vi "del2.vi"() -> ()   [LabVIEW 2025]
uses:
  Table_Filtering/Table_Filtering.lvlib
panel:
  in  "stop":bool
  out "Dataframe":string[][](array[string])
  out "Packets":string[][](table)=[["10", "11/14/2025 1:57:47 PM", "10.0.0.1", "10.0.0.2", "UDP", "0.821211", "thisisdata"], ["100", "11/14/2025 1:57:47 PM", "10.0.0.1", "10.0.0.2", "UDP", "0.956516", "thisisdata"], ["1002", "11/14/2025 1:57:47 PM", "10.0.0.1", "10.0.0.2", "UDP", "0.960987", "thisisdata"], ["1007", "11/14/2025 1:57:47 PM", "10.0.0.1", "10.0.0.2", "UDP", "0.867598", "thisisdata"], ["1009", "11/14/2025 1:57:47 PM", "10.0.0.1", "10.0.0.2", "UDP", "0.839638", "thisisdata"], ["101", "11/14/2025 1:57:47 PM", "10.0.0.1", "10.0.0.2", "UDP", "0.891709", "thisisdata"], ["1012", "11/14/2025 1:57:47 PM", "10.0.0.1", "10.0.0.2", "UDP", "0.969576", "thisisdata"], ["1017", "11/14/2025 1:57:47 PM", "10.0.0.1", "10.0.0.2", "UDP", "0.871748", "thisisdata"], ["1021", "11/14/2025 1:57:47 PM", "10.0.0.1", "10.0.0.2", "UDP", "0.904588", "thisisdata"], ["1026", "11/14/2025 1:57:47 PM", "10.0.0.1", "10.0.0.2", "UDP", "0.986150", "thisisdata"], ["1027", "11/14/2025 1:57:47 PM", "10.0.0.1", "10.0.0.2", "UDP", "0.775009", "thisisdata"], ["1028", "11/14/2025 1:57:47 PM", "10.0.0.1", "10.0.0.2", "UDP", "0.817026", "thisisdata"], ["1036", "11/14/2025 1:57:47 PM", "10.0.0.1", "10.0.0.2", "UDP", "0.839495", "thisisdata"], ["1038", "11/14/2025 1:57:47 PM", "10.0.0.1", "10.0.0.2", "UDP", "0.847314", "thisisdata"], ["1044", "11/14/2025 1:57:47 PM", "10.0.0.1", "10.0.0.2", "UDP", "0.793260", "thisisdata"], ["1048", "11/14/2025 1:57:47 PM", "10.0.0.1", "10.0.0.2", "UDP", "0.742047", "thisisdata"], ["1049", "11/14/2025 1:57:47 PM", "10.0.0.1", "10.0.0.2", "UDP", "0.771430", "thisisdata"], ["1051", "11/14/2025 1:57:47 PM", "10.0.0.1", "10.0.0.2", "UDP", "0.889463", "thisisdata"], ["1052", "11/14/2025 1:57:47 PM", "10.0.0.1", "10.0.0.2", "UDP", "0.702476", "thisisdata"], ["1053", "11/14/2025 1:57:47 PM", "10.0.0.1", "10.0.0.2", "UDP", "0.943543", "thisisdata"], ["1055", "11/14/2025 1:57:47 PM", "10.0.0.1", "10.0.0.2", "UDP", "0.912358", "thisisdata"], ["1062", "11/14/2025 1:57:47 PM", "10.0.0.1", "10.0.0.2", "UDP", "0.883876", "thisisdata"], ["1065", "11/14/2025 1:57:47 PM", "10.0.0.1", "10.0.0.2", "UDP", "0.998758", "thisisdata"], ["1066", "11/14/2025 1:57:47 PM", "10.0.0.1", "10.0.0.2", "UDP", "0.980816", "thisisdata"], ["1067", "11/14/2025 1:57:47 PM", "10.0.0.1", "10.0.0.2", "UDP", "0.862874", "thisisdata"], ["1074", "11/14/2025 1:57:47 PM", "10.0.0.1", "10.0.0.2", "UDP", "0.985200", "thisisdata"], ["1075", "11/14/2025 1:57:47 PM", "10.0.0.1", "10.0.0.2", "UDP", "0.895925", "thisisdata"], ["108", "11/14/2025 1:57:47 PM", "10.0.0.1", "10.0.0.2", "UDP", "0.746068", "thisisdata"], ["1083", "11/14/2025 1:57:47 PM", "10.0.0.1", "10.0.0.2", "UDP", "0.976636", "thisisdata"], ["1084", "11/14/2025 1:57:47 PM", "10.0.0.1", "10.0.0.2", "UDP", "0.746952", "thisisdata"], ["1086", "11/14/2025 1:57:47 PM", "10.0.0.1", "10.0.0.2", "UDP", "0.772755", "thisisdata"], ["1088", "11/14/2025 1:57:47 PM", "10.0.0.1", "10.0.0.2", "UDP", "0.942784", "thisisdata"], ["1090", "11/14/2025 1:57:47 PM", "10.0.0.1", "10.0.0.2", "UDP", "0.927067", "thisisdata"], ["1092", "11/14/2025 1:57:47 PM", "10.0.0.1", "10.0.0.2", "UDP", "0.875037", "thisisdata"], ["11", "11/14/2025 1:57:47 PM", "10.0.0.1", "10.0.0.2", "UDP", "0.939175", "thisisdata"], ["1101", "11/14/2025 1:57:47 PM", "10.0.0.1", "10.0.0.2", "UDP", "0.730371", "thisisdata"], ["1102", "11/14/2025 1:57:47 PM", "10.0.0.1", "10.0.0.2", "UDP", "0.711041", "thisisdata"], ["1103", "11/14/2025 1:57:47 PM", "10.0.0.1", "10.0.0.2", "UDP", "0.802089", "thisisdata"], ["1104", "11/14/2025 1:57:47 PM", "10.0.0.1", "10.0.0.2", "UDP", "0.975316", "thisisdata"], ["1108", "11/14/2025 1:57:47 PM", "10.0.0.1", "10.0.0.2", "UDP", "0.840307", "thisisdata"], ["1111", "11/14/2025 1:57:47 PM", "10.0.0.1", "10.0.0.2", "UDP", "0.734069", "thisisdata"], ["1113", "11/14/2025 1:57:47 PM", "10.0.0.1", "10.0.0.2", "UDP", "0.897764", "thisisdata"], ["1114", "11/14/2025 1:57:47 PM", "10.0.0.1", "10.0.0.2", "UDP", "0.704577", "thisisdata"], ["1115", "11/14/2025 1:57:47 PM", "10.0.0.1", "10.0.0.2", "UDP", "0.831595", "thisisdata"], ["1123", "11/14/2025 1:57:47 PM", "10.0.0.1", "10.0.0.2", "UDP", "0.869848", "thisisdata"], ["1130", "11/14/2025 1:57:47 PM", "10.0.0.1", "10.0.0.2", "UDP", "0.848458", "thisisdata"], ["1131", "11/14/2025 1:57:47 PM", "10.0.0.1", "10.0.0.2", "UDP", "0.914476", "thisisdata"], ["1139", "11/14/2025 1:57:47 PM", "10.0.0.1", "10.0.0.2", "UDP", "0.851881", "thisisdata"], ["1142", "11/14/2025 1:57:47 PM", "10.0.0.1", "10.0.0.2", "UDP", "0.781918", "thisisdata"], ["1148", "11/14/2025 1:57:47 PM", "10.0.0.1", "10.0.0.2", "UDP", "0.839308", "thisisdata"], ["115", "11/14/2025 1:57:47 PM", "10.0.0.1", "10.0.0.2", "UDP", "0.824463", "thisisdata"], ["1153", "11/14/2025 1:57:47 PM", "10.0.0.1", "10.0.0.2", "UDP", "0.762073", "thisisdata"], ["116", "11/14/2025 1:57:47 PM", "10.0.0.1", "10.0.0.2", "UDP", "0.718284", "thisisdata"], ["1164", "11/14/2025 1:57:47 PM", "10.0.0.1", "10.0.0.2", "UDP", "0.901802", "thisisdata"], ["1165", "11/14/2025 1:57:47 PM", "10.0.0.1", "10.0.0.2", "UDP", "0.782467", "thisisdata"], ["1168", "11/14/2025 1:57:47 PM", "10.0.0.1", "10.0.0.2", "UDP", "0.901873", "thisisdata"], ["1177", "11/14/2025 1:57:47 PM", "10.0.0.1", "10.0.0.2", "UDP", "0.889595", "thisisdata"], ["118", "11/14/2025 1:57:47 PM", "10.0.0.1", "10.0.0.2", "UDP", "0.966309", "thisisdata"], ["1181", "11/14/2025 1:57:47 PM", "10.0.0.1", "10.0.0.2", "UDP", "0.741139", "thisisdata"], ["1182", "11/14/2025 1:57:47 PM", "10.0.0.1", "10.0.0.2", "UDP", "0.954023", "thisisdata"], ["1183", "11/14/2025 1:57:47 PM", "10.0.0.1", "10.0.0.2", "UDP", "0.881562", "thisisdata"], ["1184", "11/14/2025 1:57:47 PM", "10.0.0.1", "10.0.0.2", "UDP", "0.852993", "thisisdata"], ["1185", "11/14/2025 1:57:47 PM", "10.0.0.1", "10.0.0.2", "UDP", "0.885773", "thisisdata"], ["1187", "11/14/2025 1:57:47 PM", "10.0.0.1", "10.0.0.2", "UDP", "0.801737", "thisisdata"], ["1195", "11/14/2025 1:57:47 PM", "10.0.0.1", "10.0.0.2", "UDP", "0.790347", "thisisdata"], ["1196", "11/14/2025 1:57:47 PM", "10.0.0.1", "10.0.0.2", "UDP", "0.864754", "thisisdata"], ["1197", "11/14/2025 1:57:47 PM", "10.0.0.1", "10.0.0.2", "UDP", "0.709221", "thisisdata"], ["121", "11/14/2025 1:57:47 PM", "10.0.0.1", "10.0.0.2", "UDP", "0.913497", "thisisdata"], ["1211", "11/14/2025 1:57:47 PM", "10.0.0.1", "10.0.0.2", "UDP", "0.965122", "thisisdata"], ["1213", "11/14/2025 1:57:47 PM", "10.0.0.1", "10.0.0.2", "UDP", "0.973075", "thisisdata"], ["1218", "11/14/2025 1:57:47 PM", "10.0.0.1", "10.0.0.2", "UDP", "0.904226", "thisisdata"], ["1222", "11/14/2025 1:57:47 PM", "10.0.0.1", "10.0.0.2", "UDP", "0.828121", "thisisdata"], ["1225", "11/14/2025 1:57:47 PM", "10.0.0.1", "10.0.0.2", "UDP", "0.730012", "thisisdata"], ["1226", "11/14/2025 1:57:47 PM", "10.0.0.1", "10.0.0.2", "UDP", "0.762505", "thisisdata"], ["123", "11/14/2025 1:57:47 PM", "10.0.0.1", "10.0.0.2", "UDP", "0.900157", "thisisdata"], ["1230", "11/14/2025 1:57:47 PM", "10.0.0.1", "10.0.0.2", "UDP", "0.958830", "thisisdata"], ["1231", "11/14/2025 1:57:47 PM", "10.0.0.1", "10.0.0.2", "UDP", "0.727490", "thisisdata"], ["1232", "11/14/2025 1:57:47 PM", "10.0.0.1", "10.0.0.2", "UDP", "0.913030", "thisisdata"], ["1234", "11/14/2025 1:57:47 PM", "10.0.0.1", "10.0.0.2", "UDP", "0.711353", "thisisdata"], ["1237", "11/14/2025 1:57:47 PM", "10.0.0.1", "10.0.0.2", "UDP", "0.704839", "thisisdata"], ["1240", "11/14/2025 1:57:47 PM", "10.0.0.1", "10.0.0.2", "UDP", "0.808493", "thisisdata"], ["1241", "11/14/2025 1:57:47 PM", "10.0.0.1", "10.0.0.2", "UDP", "0.750334", "thisisdata"], ["1242", "11/14/2025 1:57:47 PM", "10.0.0.1", "10.0.0.2", "UDP", "0.953795", "thisisdata"], ["1243", "11/14/2025 1:57:47 PM", "10.0.0.1", "10.0.0.2", "UDP", "0.914837", "thisisdata"], ["125", "11/14/2025 1:57:47 PM", "10.0.0.1", "10.0.0.2", "UDP", "0.850827", "thisisdata"], ["1252", "11/14/2025 1:57:47 PM", "10.0.0.1", "10.0.0.2", "UDP", "0.889690", "thisisdata"], ["1253", "11/14/2025 1:57:47 PM", "10.0.0.1", "10.0.0.2", "UDP", "0.800545", "thisisdata"], ["1255", "11/14/2025 1:57:47 PM", "10.0.0.1", "10.0.0.2", "UDP", "0.813802", "thisisdata"], ["1262", "11/14/2025 1:57:47 PM", "10.0.0.1", "10.0.0.2", "UDP", "0.882839", "thisisdata"], ["1265", "11/14/2025 1:57:47 PM", "10.0.0.1", "10.0.0.2", "UDP", "0.898409", "thisisdata"], ["127", "11/14/2025 1:57:47 PM", "10.0.0.1", "10.0.0.2", "UDP", "0.713807", "thisisdata"], ["1275", "11/14/2025 1:57:47 PM", "10.0.0.1", "10.0.0.2", "UDP", "0.972156", "thisisdata"], ["1284", "11/14/2025 1:57:47 PM", "10.0.0.1", "10.0.0.2", "UDP", "0.978269", "thisisdata"], ["1289", "11/14/2025 1:57:47 PM", "10.0.0.1", "10.0.0.2", "UDP", "0.740155", "thisisdata"], ["1299", "11/14/2025 1:57:47 PM", "10.0.0.1", "10.0.0.2", "UDP", "0.953843", "thisisdata"], ["13", "11/14/2025 1:57:47 PM", "10.0.0.1", "10.0.0.2", "UDP", "0.842815", "thisisdata"], ["1301", "11/14/2025 1:57:47 PM", "10.0.0.1", "10.0.0.2", "UDP", "0.879611", "thisisdata"], ["1302", "11/14/2025 1:57:47 PM", "10.0.0.1", "10.0.0.2", "UDP", "0.945983", "thisisdata"], ["1303", "11/14/2025 1:57:47 PM", "10.0.0.1", "10.0.0.2", "UDP", "0.755170", "thisisdata"], ["1307", "11/14/2025 1:57:47 PM", "10.0.0.1", "10.0.0.2", "UDP", "0.773780", "thisisdata"], ["1312", "11/14/2025 1:57:47 PM", "10.0.0.1", "10.0.0.2", "UDP", "0.814087", "thisisdata"], ["1314", "11/14/2025 1:57:47 PM", "10.0.0.1", "10.0.0.2", "UDP", "0.980063", "thisisdata"], ["1317", "11/14/2025 1:57:47 PM", "10.0.0.1", "10.0.0.2", "UDP", "0.829011", "thisisdata"], ["1320", "11/14/2025 1:57:47 PM", "10.0.0.1", "10.0.0.2", "UDP", "0.758120", "thisisdata"], ["1321", "11/14/2025 1:57:47 PM", "10.0.0.1", "10.0.0.2", "UDP", "0.759463", "thisisdata"], ["1322", "11/14/2025 1:57:47 PM", "10.0.0.1", "10.0.0.2", "UDP", "0.824116", "thisisdata"], ["1323", "11/14/2025 1:57:47 PM", "10.0.0.1", "10.0.0.2", "UDP", "0.762172", "thisisdata"], ["1324", "11/14/2025 1:57:47 PM", "10.0.0.1", "10.0.0.2", "UDP", "0.885589", "thisisdata"], ["1330", "11/14/2025 1:57:47 PM", "10.0.0.1", "10.0.0.2", "UDP", "0.942420", "thisisdata"], ["1333", "11/14/2025 1:57:47 PM", "10.0.0.1", "10.0.0.2", "UDP", "0.798878", "thisisdata"], ["1338", "11/14/2025 1:57:47 PM", "10.0.0.1", "10.0.0.2", "UDP", "0.748441", "thisisdata"], ["134", "11/14/2025 1:57:47 PM", "10.0.0.1", "10.0.0.2", "UDP", "0.739118", "thisisdata"], ["1341", "11/14/2025 1:57:47 PM", "10.0.0.1", "10.0.0.2", "UDP", "0.912641", "thisisdata"], ["1342", "11/14/2025 1:57:47 PM", "10.0.0.1", "10.0.0.2", "UDP", "0.833794", "thisisdata"], ["1346", "11/14/2025 1:57:47 PM", "10.0.0.1", "10.0.0.2", "UDP", "0.938173", "thisisdata"], ["1348", "11/14/2025 1:57:47 PM", "10.0.0.1", "10.0.0.2", "UDP", "0.703225", "thisisdata"], ["1349", "11/14/2025 1:57:47 PM", "10.0.0.1", "10.0.0.2", "UDP", "0.962230", "thisisdata"], ["1351", "11/14/2025 1:57:47 PM", "10.0.0.1", "10.0.0.2", "UDP", "0.923262", "thisisdata"], ["1357", "11/14/2025 1:57:47 PM", "10.0.0.1", "10.0.0.2", "UDP", "0.977014", "thisisdata"], ["1358", "11/14/2025 1:57:47 PM", "10.0.0.1", "10.0.0.2", "UDP", "0.904471", "thisisdata"], ["1360", "11/14/2025 1:57:47 PM", "10.0.0.1", "10.0.0.2", "UDP", "0.840541", "thisisdata"], ["1364", "11/14/2025 1:57:47 PM", "10.0.0.1", "10.0.0.2", "UDP", "0.759527", "thisisdata"], ["1367", "11/14/2025 1:57:47 PM", "10.0.0.1", "10.0.0.2", "UDP", "0.926483", "thisisdata"], ["1369", "11/14/2025 1:57:47 PM", "10.0.0.1", "10.0.0.2", "UDP", "0.897696", "thisisdata"], ["1371", "11/14/2025 1:57:47 PM", "10.0.0.1", "10.0.0.2", "UDP", "0.987694", "thisisdata"], ["1374", "11/14/2025 1:57:47 PM", "10.0.0.1", "10.0.0.2", "UDP", "0.795706", "thisisdata"], ["1377", "11/14/2025 1:57:47 PM", "10.0.0.1", "10.0.0.2", "UDP", "0.927883", "thisisdata"], ["1378", "11/14/2025 1:57:47 PM", "10.0.0.1", "10.0.0.2", "UDP", "0.986175", "thisisdata"], ["1379", "11/14/2025 1:57:47 PM", "10.0.0.1", "10.0.0.2", "UDP", "0.716053", "thisisdata"], ["138", "11/14/2025 1:57:47 PM", "10.0.0.1", "10.0.0.2", "UDP", "0.961495", "thisisdata"], ["1381", "11/14/2025 1:57:47 PM", "10.0.0.1", "10.0.0.2", "UDP", "0.839552", "thisisdata"], ["1382", "11/14/2025 1:57:47 PM", "10.0.0.1", "10.0.0.2", "UDP", "0.914187", "thisisdata"], ["1388", "11/14/2025 1:57:47 PM", "10.0.0.1", "10.0.0.2", "UDP", "0.890783", "thisisdata"], ["1390", "11/14/2025 1:57:47 PM", "10.0.0.1", "10.0.0.2", "UDP", "0.913426", "thisisdata"], ["1391", "11/14/2025 1:57:47 PM", "10.0.0.1", "10.0.0.2", "UDP", "0.758421", "thisisdata"], ["1394", "11/14/2025 1:57:47 PM", "10.0.0.1", "10.0.0.2", "UDP", "0.884168", "thisisdata"], ["1395", "11/14/2025 1:57:47 PM", "10.0.0.1", "10.0.0.2", "UDP", "0.773979", "thisisdata"], ["1397", "11/14/2025 1:57:47 PM", "10.0.0.1", "10.0.0.2", "UDP", "0.827235", "thisisdata"], ["14", "11/14/2025 1:57:47 PM", "10.0.0.1", "10.0.0.2", "UDP", "0.839466", "thisisdata"], ["1403", "11/14/2025 1:57:47 PM", "10.0.0.1", "10.0.0.2", "UDP", "0.889704", "thisisdata"], ["1411", "11/14/2025 1:57:47 PM", "10.0.0.1", "10.0.0.2", "UDP", "0.967881", "thisisdata"], ["1417", "11/14/2025 1:57:47 PM", "10.0.0.1", "10.0.0.2", "UDP", "0.962037", "thisisdata"], ["1418", "11/14/2025 1:57:47 PM", "10.0.0.1", "10.0.0.2", "UDP", "0.951923", "thisisdata"], ["1419", "11/14/2025 1:57:47 PM", "10.0.0.1", "10.0.0.2", "UDP", "0.912131", "thisisdata"], ["142", "11/14/2025 1:57:47 PM", "10.0.0.1", "10.0.0.2", "UDP", "0.900485", "thisisdata"], ["1421", "11/14/2025 1:57:47 PM", "10.0.0.1", "10.0.0.2", "UDP", "0.972293", "thisisdata"], ["1428", "11/14/2025 1:57:47 PM", "10.0.0.1", "10.0.0.2", "UDP", "0.706623", "thisisdata"], ["143", "11/14/2025 1:57:47 PM", "10.0.0.1", "10.0.0.2", "UDP", "0.862774", "thisisdata"], ["1430", "11/14/2025 1:57:47 PM", "10.0.0.1", "10.0.0.2", "UDP", "0.831932", "thisisdata"], ["1432", "11/14/2025 1:57:47 PM", "10.0.0.1", "10.0.0.2", "UDP", "0.955880", "thisisdata"], ["1434", "11/14/2025 1:57:47 PM", "10.0.0.1", "10.0.0.2", "UDP", "0.885487", "thisisdata"], ["1436", "11/14/2025 1:57:47 PM", "10.0.0.1", "10.0.0.2", "UDP", "0.804128", "thisisdata"], ["144", "11/14/2025 1:57:47 PM", "10.0.0.1", "10.0.0.2", "UDP", "0.837449", "thisisdata"], ["1440", "11/14/2025 1:57:47 PM", "10.0.0.1", "10.0.0.2", "UDP", "0.973148", "thisisdata"], ["1447", "11/14/2025 1:57:47 PM", "10.0.0.1", "10.0.0.2", "UDP", "0.718230", "thisisdata"], ["1449", "11/14/2025 1:57:47 PM", "10.0.0.1", "10.0.0.2", "UDP", "0.724932", "thisisdata"], ["145", "11/14/2025 1:57:47 PM", "10.0.0.1", "10.0.0.2", "UDP", "0.834936", "thisisdata"], ["1453", "11/14/2025 1:57:47 PM", "10.0.0.1", "10.0.0.2", "UDP", "0.709100", "thisisdata"], ["1457", "11/14/2025 1:57:47 PM", "10.0.0.1", "10.0.0.2", "UDP", "0.785225", "thisisdata"], ["146", "11/14/2025 1:57:47 PM", "10.0.0.1", "10.0.0.2", "UDP", "0.967161", "thisisdata"], ["1467", "11/14/2025 1:57:47 PM", "10.0.0.1", "10.0.0.2", "UDP", "0.721965", "thisisdata"], ["1468", "11/14/2025 1:57:47 PM", "10.0.0.1", "10.0.0.2", "UDP", "0.994270", "thisisdata"], ["1469", "11/14/2025 1:57:47 PM", "10.0.0.1", "10.0.0.2", "UDP", "0.848087", "thisisdata"], ["147", "11/14/2025 1:57:47 PM", "10.0.0.1", "10.0.0.2", "UDP", "0.777765", "thisisdata"], ["1473", "11/14/2025 1:57:47 PM", "10.0.0.1", "10.0.0.2", "UDP", "0.959502", "thisisdata"], ["1474", "11/14/2025 1:57:47 PM", "10.0.0.1", "10.0.0.2", "UDP", "0.934426", "thisisdata"], ["1475", "11/14/2025 1:57:47 PM", "10.0.0.1", "10.0.0.2", "UDP", "0.755909", "thisisdata"], ["1480", "11/14/2025 1:57:47 PM", "10.0.0.1", "10.0.0.2", "UDP", "0.947402", "thisisdata"], ["1482", "11/14/2025 1:57:47 PM", "10.0.0.1", "10.0.0.2", "UDP", "0.966904", "thisisdata"], ["1488", "11/14/2025 1:57:47 PM", "10.0.0.1", "10.0.0.2", "UDP", "0.717426", "thisisdata"], ["1494", "11/14/2025 1:57:47 PM", "10.0.0.1", "10.0.0.2", "UDP", "0.937831", "thisisdata"], ["1496", "11/14/2025 1:57:47 PM", "10.0.0.1", "10.0.0.2", "UDP", "0.872401", "thisisdata"], ["1497", "11/14/2025 1:57:47 PM", "10.0.0.1", "10.0.0.2", "UDP", "0.814240", "thisisdata"], ["1498", "11/14/2025 1:57:47 PM", "10.0.0.1", "10.0.0.2", "UDP", "0.750281", "thisisdata"], ["151", "11/14/2025 1:57:47 PM", "10.0.0.1", "10.0.0.2", "UDP", "0.875864", "thisisdata"], ["152", "11/14/2025 1:57:47 PM", "10.0.0.1", "10.0.0.2", "UDP", "0.771317", "thisisdata"], ["153", "11/14/2025 1:57:47 PM", "10.0.0.1", "10.0.0.2", "UDP", "0.839422", "thisisdata"], ["156", "11/14/2025 1:57:47 PM", "10.0.0.1", "10.0.0.2", "UDP", "0.729712", "thisisdata"], ["158", "11/14/2025 1:57:47 PM", "10.0.0.1", "10.0.0.2", "UDP", "0.878224", "thisisdata"], ["159", "11/14/2025 1:57:47 PM", "10.0.0.1", "10.0.0.2", "UDP", "0.963331", "thisisdata"], ["16", "11/14/2025 1:57:47 PM", "10.0.0.1", "10.0.0.2", "UDP", "0.706402", "thisisdata"], ["160", "11/14/2025 1:57:47 PM", "10.0.0.1", "10.0.0.2", "UDP", "0.803364", "thisisdata"], ["161", "11/14/2025 1:57:47 PM", "10.0.0.1", "10.0.0.2", "UDP", "0.841035", "thisisdata"], ["162", "11/14/2025 1:57:47 PM", "10.0.0.1", "10.0.0.2", "UDP", "0.815937", "thisisdata"], ["171", "11/14/2025 1:57:47 PM", "10.0.0.1", "10.0.0.2", "UDP", "0.923770", "thisisdata"], ["175", "11/14/2025 1:57:47 PM", "10.0.0.1", "10.0.0.2", "UDP", "0.775138", "thisisdata"], ["182", "11/14/2025 1:57:47 PM", "10.0.0.1", "10.0.0.2", "UDP", "0.769656", "thisisdata"], ["183", "11/14/2025 1:57:47 PM", "10.0.0.1", "10.0.0.2", "UDP", "0.886119", "thisisdata"], ["184", "11/14/2025 1:57:47 PM", "10.0.0.1", "10.0.0.2", "UDP", "0.717707", "thisisdata"], ["186", "11/14/2025 1:57:47 PM", "10.0.0.1", "10.0.0.2", "UDP", "0.963742", "thisisdata"], ["189", "11/14/2025 1:57:47 PM", "10.0.0.1", "10.0.0.2", "UDP", "0.822883", "thisisdata"], ["204", "11/14/2025 1:57:47 PM", "10.0.0.1", "10.0.0.2", "UDP", "0.812997", "thisisdata"], ["211", "11/14/2025 1:57:47 PM", "10.0.0.1", "10.0.0.2", "UDP", "0.819247", "thisisdata"], ["215", "11/14/2025 1:57:47 PM", "10.0.0.1", "10.0.0.2", "UDP", "0.723501", "thisisdata"], ["218", "11/14/2025 1:57:47 PM", "10.0.0.1", "10.0.0.2", "UDP", "0.817730", "thisisdata"], ["222", "11/14/2025 1:57:47 PM", "10.0.0.1", "10.0.0.2", "UDP", "0.952346", "thisisdata"], ["225", "11/14/2025 1:57:47 PM", "10.0.0.1", "10.0.0.2", "UDP", "0.939892", "thisisdata"], ["226", "11/14/2025 1:57:47 PM", "10.0.0.1", "10.0.0.2", "UDP", "0.992709", "thisisdata"], ["235", "11/14/2025 1:57:47 PM", "10.0.0.1", "10.0.0.2", "UDP", "0.941276", "thisisdata"], ["246", "11/14/2025 1:57:47 PM", "10.0.0.1", "10.0.0.2", "UDP", "0.904690", "thisisdata"], ["25", "11/14/2025 1:57:47 PM", "10.0.0.1", "10.0.0.2", "UDP", "0.910103", "thisisdata"], ["251", "11/14/2025 1:57:47 PM", "10.0.0.1", "10.0.0.2", "UDP", "0.720603", "thisisdata"], ["252", "11/14/2025 1:57:47 PM", "10.0.0.1", "10.0.0.2", "UDP", "0.978412", "thisisdata"], ["253", "11/14/2025 1:57:47 PM", "10.0.0.1", "10.0.0.2", "UDP", "0.859802", "thisisdata"], ["257", "11/14/2025 1:57:47 PM", "10.0.0.1", "10.0.0.2", "UDP", "0.706716", "thisisdata"], ["265", "11/14/2025 1:57:47 PM", "10.0.0.1", "10.0.0.2", "UDP", "0.954216", "thisisdata"], ["266", "11/14/2025 1:57:47 PM", "10.0.0.1", "10.0.0.2", "UDP", "0.978586", "thisisdata"], ["268", "11/14/2025 1:57:47 PM", "10.0.0.1", "10.0.0.2", "UDP", "0.728359", "thisisdata"], ["269", "11/14/2025 1:57:47 PM", "10.0.0.1", "10.0.0.2", "UDP", "0.805801", "thisisdata"], ["27", "11/14/2025 1:57:47 PM", "10.0.0.1", "10.0.0.2", "UDP", "0.890670", "thisisdata"], ["270", "11/14/2025 1:57:47 PM", "10.0.0.1", "10.0.0.2", "UDP", "0.730876", "thisisdata"], ["271", "11/14/2025 1:57:47 PM", "10.0.0.1", "10.0.0.2", "UDP", "0.964321", "thisisdata"], ["273", "11/14/2025 1:57:47 PM", "10.0.0.1", "10.0.0.2", "UDP", "0.822445", "thisisdata"], ["280", "11/14/2025 1:57:47 PM", "10.0.0.1", "10.0.0.2", "UDP", "0.805915", "thisisdata"], ["282", "11/14/2025 1:57:47 PM", "10.0.0.1", "10.0.0.2", "UDP", "0.995119", "thisisdata"], ["285", "11/14/2025 1:57:47 PM", "10.0.0.1", "10.0.0.2", "UDP", "0.702493", "thisisdata"], ["287", "11/14/2025 1:57:47 PM", "10.0.0.1", "10.0.0.2", "UDP", "0.895930", "thisisdata"], ["293", "11/14/2025 1:57:47 PM", "10.0.0.1", "10.0.0.2", "UDP", "0.782899", "thisisdata"], ["30", "11/14/2025 1:57:47 PM", "10.0.0.1", "10.0.0.2", "UDP", "0.919602", "thisisdata"], ["302", "11/14/2025 1:57:47 PM", "10.0.0.1", "10.0.0.2", "UDP", "0.702472", "thisisdata"], ["303", "11/14/2025 1:57:47 PM", "10.0.0.1", "10.0.0.2", "UDP", "0.776732", "thisisdata"], ["304", "11/14/2025 1:57:47 PM", "10.0.0.1", "10.0.0.2", "UDP", "0.805126", "thisisdata"], ["305", "11/14/2025 1:57:47 PM", "10.0.0.1", "10.0.0.2", "UDP", "0.974208", "thisisdata"], ["306", "11/14/2025 1:57:47 PM", "10.0.0.1", "10.0.0.2", "UDP", "0.799271", "thisisdata"], ["307", "11/14/2025 1:57:47 PM", "10.0.0.1", "10.0.0.2", "UDP", "0.985518", "thisisdata"], ["310", "11/14/2025 1:57:47 PM", "10.0.0.1", "10.0.0.2", "UDP", "0.995978", "thisisdata"], ["311", "11/14/2025 1:57:47 PM", "10.0.0.1", "10.0.0.2", "UDP", "0.987227", "thisisdata"], ["312", "11/14/2025 1:57:47 PM", "10.0.0.1", "10.0.0.2", "UDP", "0.797511", "thisisdata"], ["314", "11/14/2025 1:57:47 PM", "10.0.0.1", "10.0.0.2", "UDP", "0.838158", "thisisdata"], ["316", "11/14/2025 1:57:47 PM", "10.0.0.1", "10.0.0.2", "UDP", "0.898183", "thisisdata"], ["319", "11/14/2025 1:57:47 PM", "10.0.0.1", "10.0.0.2", "UDP", "0.813462", "thisisdata"], ["320", "11/14/2025 1:57:47 PM", "10.0.0.1", "10.0.0.2", "UDP", "0.725049", "thisisdata"], ["322", "11/14/2025 1:57:47 PM", "10.0.0.1", "10.0.0.2", "UDP", "0.954221", "thisisdata"], ["324", "11/14/2025 1:57:47 PM", "10.0.0.1", "10.0.0.2", "UDP", "0.773913", "thisisdata"], ["330", "11/14/2025 1:57:47 PM", "10.0.0.1", "10.0.0.2", "UDP", "0.846395", "thisisdata"], ["331", "11/14/2025 1:57:47 PM", "10.0.0.1", "10.0.0.2", "UDP", "0.868667", "thisisdata"], ["333", "11/14/2025 1:57:47 PM", "10.0.0.1", "10.0.0.2", "UDP", "0.915934", "thisisdata"], ["335", "11/14/2025 1:57:47 PM", "10.0.0.1", "10.0.0.2", "UDP", "0.744820", "thisisdata"], ["344", "11/14/2025 1:57:47 PM", "10.0.0.1", "10.0.0.2", "UDP", "0.737303", "thisisdata"], ["345", "11/14/2025 1:57:47 PM", "10.0.0.1", "10.0.0.2", "UDP", "0.744197", "thisisdata"], ["347", "11/14/2025 1:57:47 PM", "10.0.0.1", "10.0.0.2", "UDP", "0.816133", "thisisdata"], ["35", "11/14/2025 1:57:47 PM", "10.0.0.1", "10.0.0.2", "UDP", "0.980754", "thisisdata"], ["359", "11/14/2025 1:57:47 PM", "10.0.0.1", "10.0.0.2", "UDP", "0.710696", "thisisdata"], ["36", "11/14/2025 1:57:47 PM", "10.0.0.1", "10.0.0.2", "UDP", "0.821418", "thisisdata"], ["361", "11/14/2025 1:57:47 PM", "10.0.0.1", "10.0.0.2", "UDP", "0.810013", "thisisdata"], ["369", "11/14/2025 1:57:47 PM", "10.0.0.1", "10.0.0.2", "UDP", "0.918693", "thisisdata"], ["373", "11/14/2025 1:57:47 PM", "10.0.0.1", "10.0.0.2", "UDP", "0.860255", "thisisdata"], ["376", "11/14/2025 1:57:47 PM", "10.0.0.1", "10.0.0.2", "UDP", "0.749631", "thisisdata"], ["38", "11/14/2025 1:57:47 PM", "10.0.0.1", "10.0.0.2", "UDP", "0.844976", "thisisdata"], ["383", "11/14/2025 1:57:47 PM", "10.0.0.1", "10.0.0.2", "UDP", "0.800813", "thisisdata"], ["384", "11/14/2025 1:57:47 PM", "10.0.0.1", "10.0.0.2", "UDP", "0.765681", "thisisdata"], ["391", "11/14/2025 1:57:47 PM", "10.0.0.1", "10.0.0.2", "UDP", "0.710353", "thisisdata"], ["392", "11/14/2025 1:57:47 PM", "10.0.0.1", "10.0.0.2", "UDP", "0.798826", "thisisdata"], ["393", "11/14/2025 1:57:47 PM", "10.0.0.1", "10.0.0.2", "UDP", "0.888259", "thisisdata"], ["394", "11/14/2025 1:57:47 PM", "10.0.0.1", "10.0.0.2", "UDP", "0.728993", "thisisdata"], ["406", "11/14/2025 1:57:47 PM", "10.0.0.1", "10.0.0.2", "UDP", "0.924575", "thisisdata"], ["408", "11/14/2025 1:57:47 PM", "10.0.0.1", "10.0.0.2", "UDP", "0.827347", "thisisdata"], ["41", "11/14/2025 1:57:47 PM", "10.0.0.1", "10.0.0.2", "UDP", "0.897112", "thisisdata"], ["412", "11/14/2025 1:57:47 PM", "10.0.0.1", "10.0.0.2", "UDP", "0.823947", "thisisdata"], ["414", "11/14/2025 1:57:47 PM", "10.0.0.1", "10.0.0.2", "UDP", "0.706129", "thisisdata"], ["415", "11/14/2025 1:57:47 PM", "10.0.0.1", "10.0.0.2", "UDP", "0.712052", "thisisdata"], ["42", "11/14/2025 1:57:47 PM", "10.0.0.1", "10.0.0.2", "UDP", "0.984320", "thisisdata"], ["421", "11/14/2025 1:57:47 PM", "10.0.0.1", "10.0.0.2", "UDP", "0.790512", "thisisdata"], ["428", "11/14/2025 1:57:47 PM", "10.0.0.1", "10.0.0.2", "UDP", "0.825226", "thisisdata"], ["431", "11/14/2025 1:57:47 PM", "10.0.0.1", "10.0.0.2", "UDP", "0.866616", "thisisdata"], ["433", "11/14/2025 1:57:47 PM", "10.0.0.1", "10.0.0.2", "UDP", "0.906895", "thisisdata"], ["442", "11/14/2025 1:57:47 PM", "10.0.0.1", "10.0.0.2", "UDP", "0.885974", "thisisdata"], ["448", "11/14/2025 1:57:47 PM", "10.0.0.1", "10.0.0.2", "UDP", "0.888818", "thisisdata"], ["453", "11/14/2025 1:57:47 PM", "10.0.0.1", "10.0.0.2", "UDP", "0.742889", "thisisdata"], ["456", "11/14/2025 1:57:47 PM", "10.0.0.1", "10.0.0.2", "UDP", "0.808371", "thisisdata"], ["459", "11/14/2025 1:57:47 PM", "10.0.0.1", "10.0.0.2", "UDP", "0.878908", "thisisdata"], ["461", "11/14/2025 1:57:47 PM", "10.0.0.1", "10.0.0.2", "UDP", "0.935594", "thisisdata"], ["463", "11/14/2025 1:57:47 PM", "10.0.0.1", "10.0.0.2", "UDP", "0.917788", "thisisdata"], ["465", "11/14/2025 1:57:47 PM", "10.0.0.1", "10.0.0.2", "UDP", "0.924728", "thisisdata"], ["467", "11/14/2025 1:57:47 PM", "10.0.0.1", "10.0.0.2", "UDP", "0.802965", "thisisdata"], ["471", "11/14/2025 1:57:47 PM", "10.0.0.1", "10.0.0.2", "UDP", "0.920198", "thisisdata"], ["473", "11/14/2025 1:57:47 PM", "10.0.0.1", "10.0.0.2", "UDP", "0.712752", "thisisdata"], ["48", "11/14/2025 1:57:47 PM", "10.0.0.1", "10.0.0.2", "UDP", "0.894854", "thisisdata"], ["484", "11/14/2025 1:57:47 PM", "10.0.0.1", "10.0.0.2", "UDP", "0.934918", "thisisdata"], ["487", "11/14/2025 1:57:47 PM", "10.0.0.1", "10.0.0.2", "UDP", "0.753021", "thisisdata"], ["489", "11/14/2025 1:57:47 PM", "10.0.0.1", "10.0.0.2", "UDP", "0.794461", "thisisdata"], ["493", "11/14/2025 1:57:47 PM", "10.0.0.1", "10.0.0.2", "UDP", "0.879307", "thisisdata"], ["494", "11/14/2025 1:57:47 PM", "10.0.0.1", "10.0.0.2", "UDP", "0.821176", "thisisdata"], ["496", "11/14/2025 1:57:47 PM", "10.0.0.1", "10.0.0.2", "UDP", "0.808411", "thisisdata"], ["498", "11/14/2025 1:57:47 PM", "10.0.0.1", "10.0.0.2", "UDP", "0.911798", "thisisdata"], ["5", "11/14/2025 1:57:47 PM", "10.0.0.1", "10.0.0.2", "UDP", "0.924127", "thisisdata"], ["501", "11/14/2025 1:57:47 PM", "10.0.0.1", "10.0.0.2", "UDP", "0.946039", "thisisdata"], ["505", "11/14/2025 1:57:47 PM", "10.0.0.1", "10.0.0.2", "UDP", "0.800570", "thisisdata"], ["509", "11/14/2025 1:57:47 PM", "10.0.0.1", "10.0.0.2", "UDP", "0.879202", "thisisdata"], ["511", "11/14/2025 1:57:47 PM", "10.0.0.1", "10.0.0.2", "UDP", "0.707965", "thisisdata"], ["517", "11/14/2025 1:57:47 PM", "10.0.0.1", "10.0.0.2", "UDP", "0.759952", "thisisdata"], ["518", "11/14/2025 1:57:47 PM", "10.0.0.1", "10.0.0.2", "UDP", "0.720618", "thisisdata"], ["520", "11/14/2025 1:57:47 PM", "10.0.0.1", "10.0.0.2", "UDP", "0.806107", "thisisdata"], ["530", "11/14/2025 1:57:47 PM", "10.0.0.1", "10.0.0.2", "UDP", "0.995294", "thisisdata"], ["531", "11/14/2025 1:57:47 PM", "10.0.0.1", "10.0.0.2", "UDP", "0.734341", "thisisdata"], ["538", "11/14/2025 1:57:47 PM", "10.0.0.1", "10.0.0.2", "UDP", "0.791430", "thisisdata"], ["552", "11/14/2025 1:57:47 PM", "10.0.0.1", "10.0.0.2", "UDP", "0.803719", "thisisdata"], ["553", "11/14/2025 1:57:47 PM", "10.0.0.1", "10.0.0.2", "UDP", "0.798672", "thisisdata"], ["555", "11/14/2025 1:57:47 PM", "10.0.0.1", "10.0.0.2", "UDP", "0.718180", "thisisdata"], ["556", "11/14/2025 1:57:47 PM", "10.0.0.1", "10.0.0.2", "UDP", "0.712425", "thisisdata"], ["557", "11/14/2025 1:57:47 PM", "10.0.0.1", "10.0.0.2", "UDP", "0.839688", "thisisdata"], ["561", "11/14/2025 1:57:47 PM", "10.0.0.1", "10.0.0.2", "UDP", "0.973886", "thisisdata"], ["575", "11/14/2025 1:57:47 PM", "10.0.0.1", "10.0.0.2", "UDP", "0.829130", "thisisdata"], ["576", "11/14/2025 1:57:47 PM", "10.0.0.1", "10.0.0.2", "UDP", "0.725344", "thisisdata"], ["579", "11/14/2025 1:57:47 PM", "10.0.0.1", "10.0.0.2", "UDP", "0.857040", "thisisdata"], ["580", "11/14/2025 1:57:47 PM", "10.0.0.1", "10.0.0.2", "UDP", "0.919608", "thisisdata"], ["584", "11/14/2025 1:57:47 PM", "10.0.0.1", "10.0.0.2", "UDP", "0.875136", "thisisdata"], ["585", "11/14/2025 1:57:47 PM", "10.0.0.1", "10.0.0.2", "UDP", "0.791057", "thisisdata"], ["59", "11/14/2025 1:57:47 PM", "10.0.0.1", "10.0.0.2", "UDP", "0.836493", "thisisdata"], ["591", "11/14/2025 1:57:47 PM", "10.0.0.1", "10.0.0.2", "UDP", "0.861319", "thisisdata"], ["592", "11/14/2025 1:57:47 PM", "10.0.0.1", "10.0.0.2", "UDP", "0.916902", "thisisdata"], ["599", "11/14/2025 1:57:47 PM", "10.0.0.1", "10.0.0.2", "UDP", "0.903742", "thisisdata"], ["60", "11/14/2025 1:57:47 PM", "10.0.0.1", "10.0.0.2", "UDP", "0.871553", "thisisdata"], ["603", "11/14/2025 1:57:47 PM", "10.0.0.1", "10.0.0.2", "UDP", "0.905091", "thisisdata"], ["606", "11/14/2025 1:57:47 PM", "10.0.0.1", "10.0.0.2", "UDP", "0.886018", "thisisdata"], ["609", "11/14/2025 1:57:47 PM", "10.0.0.1", "10.0.0.2", "UDP", "0.710266", "thisisdata"], ["610", "11/14/2025 1:57:47 PM", "10.0.0.1", "10.0.0.2", "UDP", "0.785021", "thisisdata"], ["614", "11/14/2025 1:57:47 PM", "10.0.0.1", "10.0.0.2", "UDP", "0.714634", "thisisdata"], ["622", "11/14/2025 1:57:47 PM", "10.0.0.1", "10.0.0.2", "UDP", "0.912282", "thisisdata"], ["624", "11/14/2025 1:57:47 PM", "10.0.0.1", "10.0.0.2", "UDP", "0.890598", "thisisdata"], ["631", "11/14/2025 1:57:47 PM", "10.0.0.1", "10.0.0.2", "UDP", "0.748006", "thisisdata"], ["634", "11/14/2025 1:57:47 PM", "10.0.0.1", "10.0.0.2", "UDP", "0.791920", "thisisdata"], ["64", "11/14/2025 1:57:47 PM", "10.0.0.1", "10.0.0.2", "UDP", "0.967066", "thisisdata"], ["642", "11/14/2025 1:57:47 PM", "10.0.0.1", "10.0.0.2", "UDP", "0.783278", "thisisdata"], ["644", "11/14/2025 1:57:47 PM", "10.0.0.1", "10.0.0.2", "UDP", "0.893851", "thisisdata"], ["65", "11/14/2025 1:57:47 PM", "10.0.0.1", "10.0.0.2", "UDP", "0.809766", "thisisdata"], ["657", "11/14/2025 1:57:47 PM", "10.0.0.1", "10.0.0.2", "UDP", "0.710376", "thisisdata"], ["660", "11/14/2025 1:57:47 PM", "10.0.0.1", "10.0.0.2", "UDP", "0.897561", "thisisdata"], ["661", "11/14/2025 1:57:47 PM", "10.0.0.1", "10.0.0.2", "UDP", "0.907407", "thisisdata"], ["668", "11/14/2025 1:57:47 PM", "10.0.0.1", "10.0.0.2", "UDP", "0.970645", "thisisdata"], ["669", "11/14/2025 1:57:47 PM", "10.0.0.1", "10.0.0.2", "UDP", "0.994801", "thisisdata"], ["671", "11/14/2025 1:57:47 PM", "10.0.0.1", "10.0.0.2", "UDP", "0.957190", "thisisdata"], ["672", "11/14/2025 1:57:47 PM", "10.0.0.1", "10.0.0.2", "UDP", "0.834875", "thisisdata"], ["683", "11/14/2025 1:57:47 PM", "10.0.0.1", "10.0.0.2", "UDP", "0.893810", "thisisdata"], ["692", "11/14/2025 1:57:47 PM", "10.0.0.1", "10.0.0.2", "UDP", "0.716870", "thisisdata"], ["698", "11/14/2025 1:57:47 PM", "10.0.0.1", "10.0.0.2", "UDP", "0.812164", "thisisdata"], ["699", "11/14/2025 1:57:47 PM", "10.0.0.1", "10.0.0.2", "UDP", "0.959842", "thisisdata"], ["700", "11/14/2025 1:57:47 PM", "10.0.0.1", "10.0.0.2", "UDP", "0.726590", "thisisdata"], ["711", "11/14/2025 1:57:47 PM", "10.0.0.1", "10.0.0.2", "UDP", "0.823803", "thisisdata"], ["714", "11/14/2025 1:57:47 PM", "10.0.0.1", "10.0.0.2", "UDP", "0.773208", "thisisdata"], ["718", "11/14/2025 1:57:47 PM", "10.0.0.1", "10.0.0.2", "UDP", "0.768409", "thisisdata"], ["721", "11/14/2025 1:57:47 PM", "10.0.0.1", "10.0.0.2", "UDP", "0.793787", "thisisdata"], ["725", "11/14/2025 1:57:47 PM", "10.0.0.1", "10.0.0.2", "UDP", "0.976198", "thisisdata"], ["730", "11/14/2025 1:57:47 PM", "10.0.0.1", "10.0.0.2", "UDP", "0.885853", "thisisdata"], ["731", "11/14/2025 1:57:47 PM", "10.0.0.1", "10.0.0.2", "UDP", "0.842282", "thisisdata"], ["734", "11/14/2025 1:57:47 PM", "10.0.0.1", "10.0.0.2", "UDP", "0.751845", "thisisdata"], ["735", "11/14/2025 1:57:47 PM", "10.0.0.1", "10.0.0.2", "UDP", "0.775000", "thisisdata"], ["739", "11/14/2025 1:57:47 PM", "10.0.0.1", "10.0.0.2", "UDP", "0.933339", "thisisdata"], ["74", "11/14/2025 1:57:47 PM", "10.0.0.1", "10.0.0.2", "UDP", "0.927019", "thisisdata"], ["740", "11/14/2025 1:57:47 PM", "10.0.0.1", "10.0.0.2", "UDP", "0.862581", "thisisdata"], ["75", "11/14/2025 1:57:47 PM", "10.0.0.1", "10.0.0.2", "UDP", "0.712333", "thisisdata"], ["752", "11/14/2025 1:57:47 PM", "10.0.0.1", "10.0.0.2", "UDP", "0.853785", "thisisdata"], ["754", "11/14/2025 1:57:47 PM", "10.0.0.1", "10.0.0.2", "UDP", "0.961801", "thisisdata"], ["756", "11/14/2025 1:57:47 PM", "10.0.0.1", "10.0.0.2", "UDP", "0.885805", "thisisdata"], ["761", "11/14/2025 1:57:47 PM", "10.0.0.1", "10.0.0.2", "UDP", "0.892997", "thisisdata"], ["762", "11/14/2025 1:57:47 PM", "10.0.0.1", "10.0.0.2", "UDP", "0.981252", "thisisdata"], ["763", "11/14/2025 1:57:47 PM", "10.0.0.1", "10.0.0.2", "UDP", "0.739524", "thisisdata"], ["779", "11/14/2025 1:57:47 PM", "10.0.0.1", "10.0.0.2", "UDP", "0.846841", "thisisdata"], ["782", "11/14/2025 1:57:47 PM", "10.0.0.1", "10.0.0.2", "UDP", "0.960776", "thisisdata"], ["784", "11/14/2025 1:57:47 PM", "10.0.0.1", "10.0.0.2", "UDP", "0.834294", "thisisdata"], ["786", "11/14/2025 1:57:47 PM", "10.0.0.1", "10.0.0.2", "UDP", "0.976165", "thisisdata"], ["794", "11/14/2025 1:57:47 PM", "10.0.0.1", "10.0.0.2", "UDP", "0.738251", "thisisdata"], ["796", "11/14/2025 1:57:47 PM", "10.0.0.1", "10.0.0.2", "UDP", "0.765415", "thisisdata"], ["80", "11/14/2025 1:57:47 PM", "10.0.0.1", "10.0.0.2", "UDP", "0.838034", "thisisdata"], ["804", "11/14/2025 1:57:47 PM", "10.0.0.1", "10.0.0.2", "UDP", "0.832158", "thisisdata"], ["806", "11/14/2025 1:57:47 PM", "10.0.0.1", "10.0.0.2", "UDP", "0.872118", "thisisdata"], ["809", "11/14/2025 1:57:47 PM", "10.0.0.1", "10.0.0.2", "UDP", "0.906668", "thisisdata"], ["811", "11/14/2025 1:57:47 PM", "10.0.0.1", "10.0.0.2", "UDP", "0.765262", "thisisdata"], ["816", "11/14/2025 1:57:47 PM", "10.0.0.1", "10.0.0.2", "UDP", "0.937976", "thisisdata"], ["832", "11/14/2025 1:57:47 PM", "10.0.0.1", "10.0.0.2", "UDP", "0.910402", "thisisdata"], ["844", "11/14/2025 1:57:47 PM", "10.0.0.1", "10.0.0.2", "UDP", "0.916379", "thisisdata"], ["847", "11/14/2025 1:57:47 PM", "10.0.0.1", "10.0.0.2", "UDP", "0.823197", "thisisdata"], ["849", "11/14/2025 1:57:47 PM", "10.0.0.1", "10.0.0.2", "UDP", "0.788440", "thisisdata"], ["851", "11/14/2025 1:57:47 PM", "10.0.0.1", "10.0.0.2", "UDP", "0.842912", "thisisdata"], ["858", "11/14/2025 1:57:47 PM", "10.0.0.1", "10.0.0.2", "UDP", "0.800903", "thisisdata"], ["859", "11/14/2025 1:57:47 PM", "10.0.0.1", "10.0.0.2", "UDP", "0.976923", "thisisdata"], ["86", "11/14/2025 1:57:47 PM", "10.0.0.1", "10.0.0.2", "UDP", "0.854198", "thisisdata"], ["861", "11/14/2025 1:57:47 PM", "10.0.0.1", "10.0.0.2", "UDP", "0.815290", "thisisdata"], ["862", "11/14/2025 1:57:47 PM", "10.0.0.1", "10.0.0.2", "UDP", "0.953745", "thisisdata"], ["863", "11/14/2025 1:57:47 PM", "10.0.0.1", "10.0.0.2", "UDP", "0.960371", "thisisdata"], ["864", "11/14/2025 1:57:47 PM", "10.0.0.1", "10.0.0.2", "UDP", "0.852174", "thisisdata"], ["865", "11/14/2025 1:57:47 PM", "10.0.0.1", "10.0.0.2", "UDP", "0.969242", "thisisdata"], ["870", "11/14/2025 1:57:47 PM", "10.0.0.1", "10.0.0.2", "UDP", "0.947803", "thisisdata"], ["871", "11/14/2025 1:57:47 PM", "10.0.0.1", "10.0.0.2", "UDP", "0.985852", "thisisdata"], ["874", "11/14/2025 1:57:47 PM", "10.0.0.1", "10.0.0.2", "UDP", "0.745448", "thisisdata"], ["879", "11/14/2025 1:57:47 PM", "10.0.0.1", "10.0.0.2", "UDP", "0.828622", "thisisdata"], ["881", "11/14/2025 1:57:47 PM", "10.0.0.1", "10.0.0.2", "UDP", "0.709092", "thisisdata"], ["882", "11/14/2025 1:57:47 PM", "10.0.0.1", "10.0.0.2", "UDP", "0.754218", "thisisdata"], ["884", "11/14/2025 1:57:47 PM", "10.0.0.1", "10.0.0.2", "UDP", "0.815853", "thisisdata"], ["887", "11/14/2025 1:57:47 PM", "10.0.0.1", "10.0.0.2", "UDP", "0.873913", "thisisdata"], ["888", "11/14/2025 1:57:47 PM", "10.0.0.1", "10.0.0.2", "UDP", "0.999693", "thisisdata"], ["889", "11/14/2025 1:57:47 PM", "10.0.0.1", "10.0.0.2", "UDP", "0.949421", "thisisdata"], ["89", "11/14/2025 1:57:47 PM", "10.0.0.1", "10.0.0.2", "UDP", "0.867253", "thisisdata"], ["897", "11/14/2025 1:57:47 PM", "10.0.0.1", "10.0.0.2", "UDP", "0.872446", "thisisdata"], ["898", "11/14/2025 1:57:47 PM", "10.0.0.1", "10.0.0.2", "UDP", "0.932192", "thisisdata"], ["899", "11/14/2025 1:57:47 PM", "10.0.0.1", "10.0.0.2", "UDP", "0.896984", "thisisdata"], ["9", "11/14/2025 1:57:47 PM", "10.0.0.1", "10.0.0.2", "UDP", "0.840249", "thisisdata"], ["909", "11/14/2025 1:57:47 PM", "10.0.0.1", "10.0.0.2", "UDP", "0.863075", "thisisdata"], ["91", "11/14/2025 1:57:47 PM", "10.0.0.1", "10.0.0.2", "UDP", "0.974346", "thisisdata"], ["913", "11/14/2025 1:57:47 PM", "10.0.0.1", "10.0.0.2", "UDP", "0.930396", "thisisdata"], ["914", "11/14/2025 1:57:47 PM", "10.0.0.1", "10.0.0.2", "UDP", "0.937608", "thisisdata"], ["918", "11/14/2025 1:57:47 PM", "10.0.0.1", "10.0.0.2", "UDP", "0.813773", "thisisdata"], ["922", "11/14/2025 1:57:47 PM", "10.0.0.1", "10.0.0.2", "UDP", "0.903496", "thisisdata"], ["925", "11/14/2025 1:57:47 PM", "10.0.0.1", "10.0.0.2", "UDP", "0.836203", "thisisdata"], ["93", "11/14/2025 1:57:47 PM", "10.0.0.1", "10.0.0.2", "UDP", "0.992103", "thisisdata"], ["931", "11/14/2025 1:57:47 PM", "10.0.0.1", "10.0.0.2", "UDP", "0.742922", "thisisdata"], ["935", "11/14/2025 1:57:47 PM", "10.0.0.1", "10.0.0.2", "UDP", "0.942935", "thisisdata"], ["936", "11/14/2025 1:57:47 PM", "10.0.0.1", "10.0.0.2", "UDP", "0.731021", "thisisdata"], ["94", "11/14/2025 1:57:47 PM", "10.0.0.1", "10.0.0.2", "UDP", "0.833321", "thisisdata"], ["944", "11/14/2025 1:57:47 PM", "10.0.0.1", "10.0.0.2", "UDP", "0.700170", "thisisdata"], ["945", "11/14/2025 1:57:47 PM", "10.0.0.1", "10.0.0.2", "UDP", "0.795369", "thisisdata"], ["946", "11/14/2025 1:57:47 PM", "10.0.0.1", "10.0.0.2", "UDP", "0.705826", "thisisdata"], ["950", "11/14/2025 1:57:47 PM", "10.0.0.1", "10.0.0.2", "UDP", "0.903245", "thisisdata"], ["956", "11/14/2025 1:57:47 PM", "10.0.0.1", "10.0.0.2", "UDP", "0.772137", "thisisdata"], ["962", "11/14/2025 1:57:47 PM", "10.0.0.1", "10.0.0.2", "UDP", "0.785660", "thisisdata"], ["971", "11/14/2025 1:57:47 PM", "10.0.0.1", "10.0.0.2", "UDP", "0.958167", "thisisdata"], ["973", "11/14/2025 1:57:47 PM", "10.0.0.1", "10.0.0.2", "UDP", "0.941597", "thisisdata"], ["974", "11/14/2025 1:57:47 PM", "10.0.0.1", "10.0.0.2", "UDP", "0.956441", "thisisdata"], ["976", "11/14/2025 1:57:47 PM", "10.0.0.1", "10.0.0.2", "UDP", "0.908337", "thisisdata"], ["977", "11/14/2025 1:57:47 PM", "10.0.0.1", "10.0.0.2", "UDP", "0.752689", "thisisdata"], ["983", "11/14/2025 1:57:47 PM", "10.0.0.1", "10.0.0.2", "UDP", "0.933649", "thisisdata"], ["985", "11/14/2025 1:57:47 PM", "10.0.0.1", "10.0.0.2", "UDP", "0.788836", "thisisdata"], ["987", "11/14/2025 1:57:47 PM", "10.0.0.1", "10.0.0.2", "UDP", "0.979633", "thisisdata"], ["988", "11/14/2025 1:57:47 PM", "10.0.0.1", "10.0.0.2", "UDP", "0.723583", "thisisdata"], ["989", "11/14/2025 1:57:47 PM", "10.0.0.1", "10.0.0.2", "UDP", "0.910875", "thisisdata"], ["99", "11/14/2025 1:57:47 PM", "10.0.0.1", "10.0.0.2", "UDP", "0.869477", "thisisdata"], ["995", "11/14/2025 1:57:47 PM", "10.0.0.1", "10.0.0.2", "UDP", "0.827503", "thisisdata"], ["996", "11/14/2025 1:57:47 PM", "10.0.0.1", "10.0.0.2", "UDP", "0.904767", "thisisdata"], ["999", "11/14/2025 1:57:47 PM", "10.0.0.1", "10.0.0.2", "UDP", "0.952043", "thisisdata"]]
  in  "Filter String":string="Protocol == UDP AND Length > 0.7 OR Source == 192.168.1.1"
  in  "Sort by":u16(ring) items=["Packet_Number", "Timestamp", "Source", "Destination", "Protocol", "Length", "Data"]
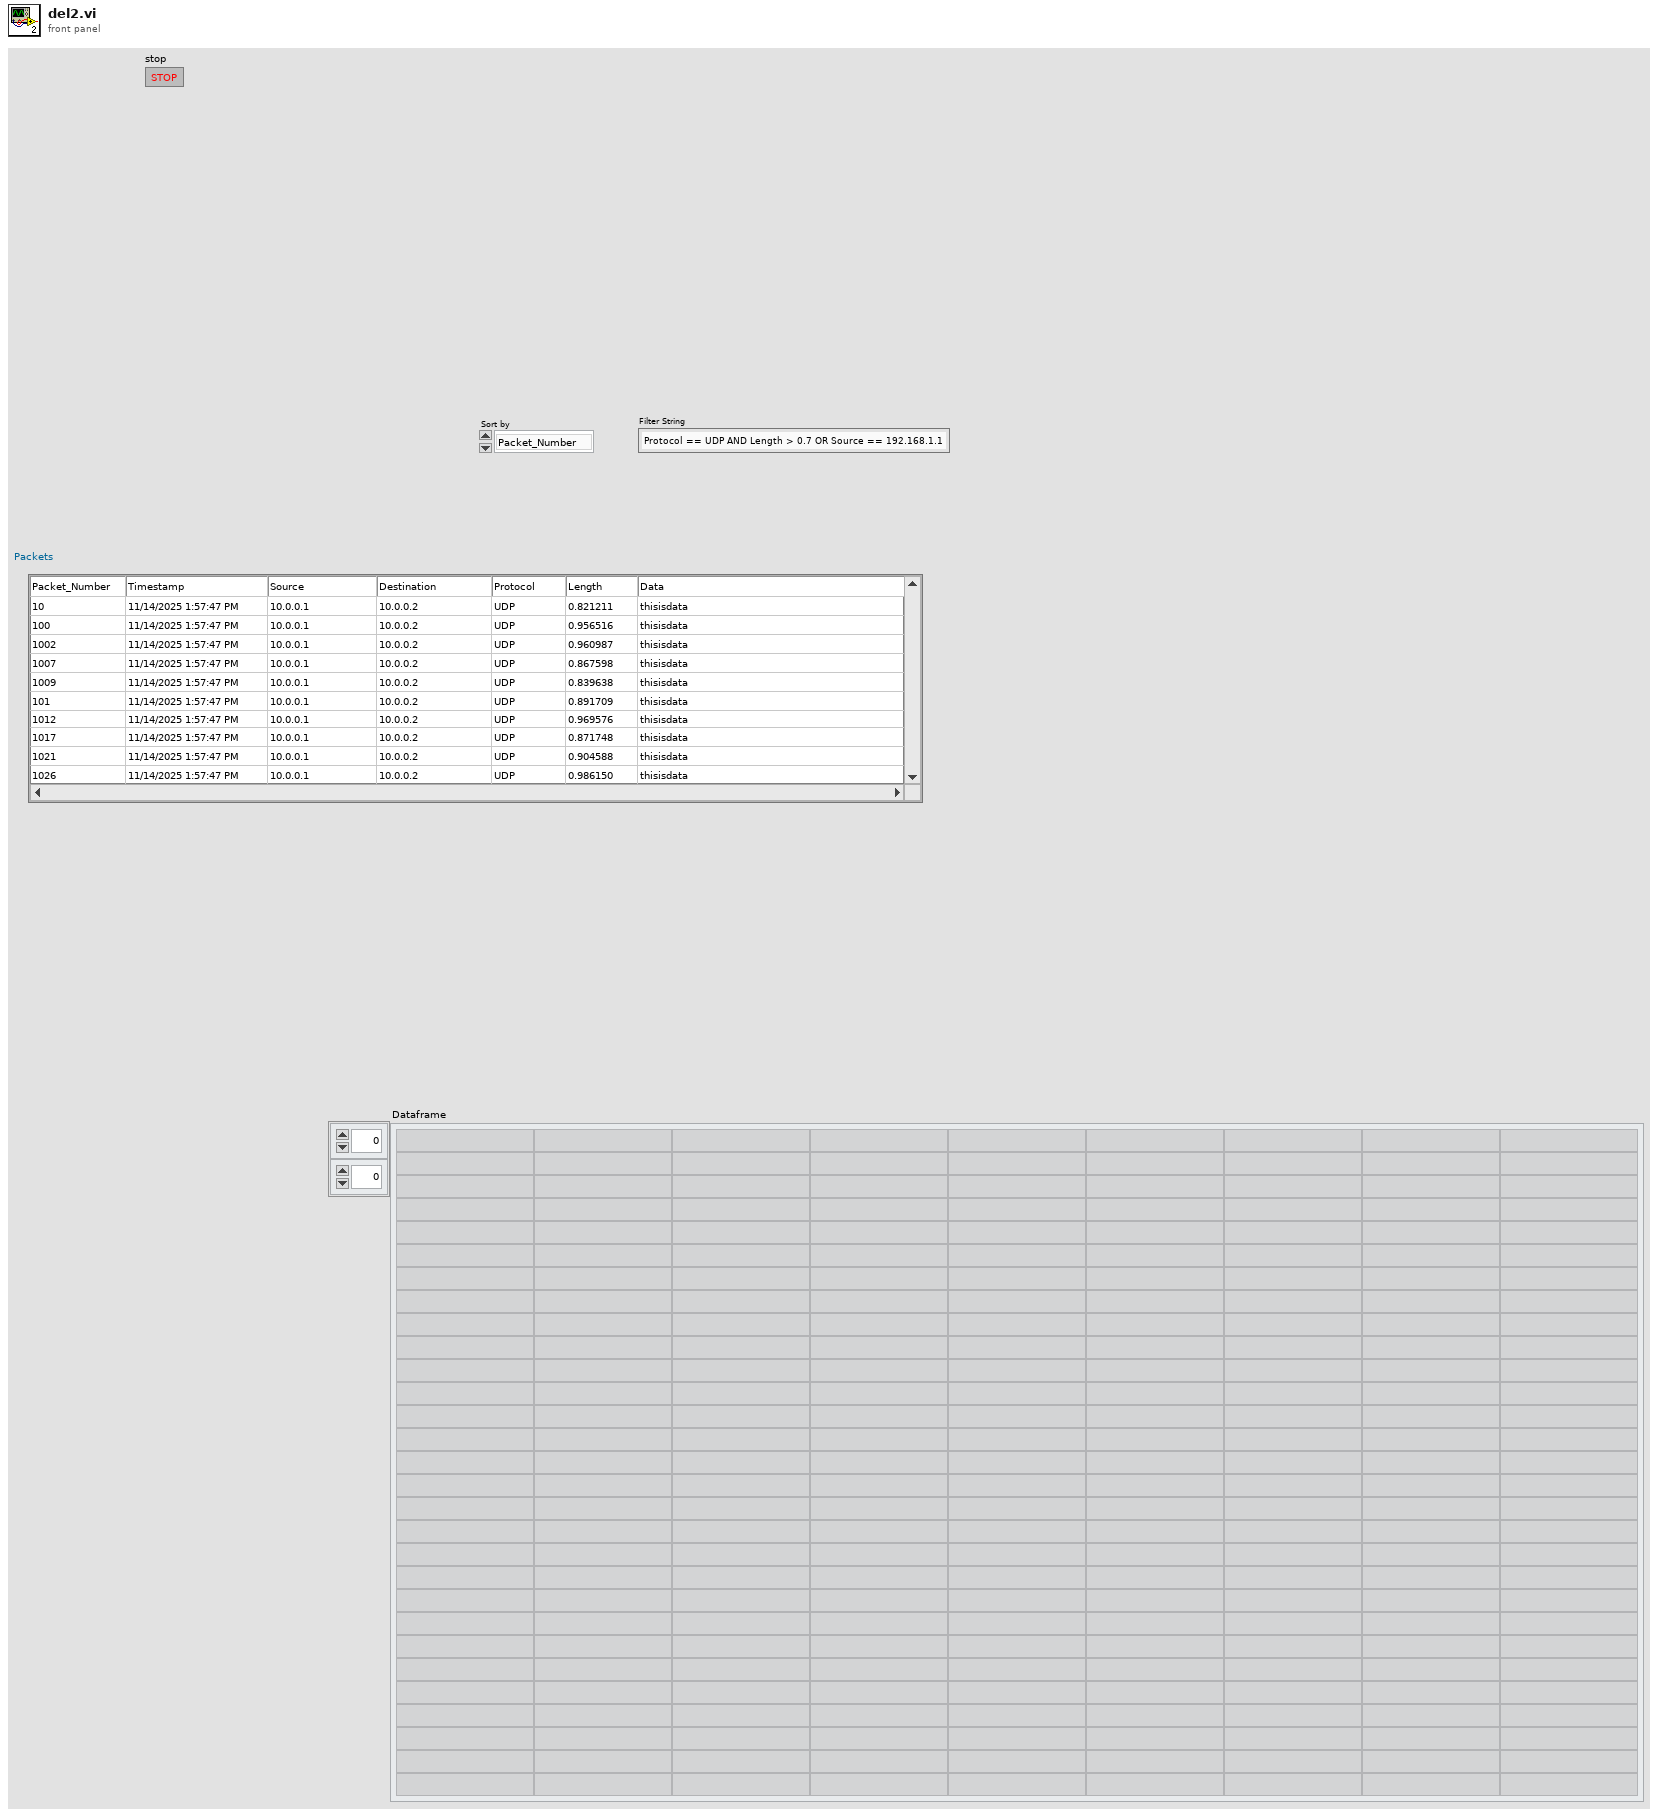
[diagram p1: front panel]
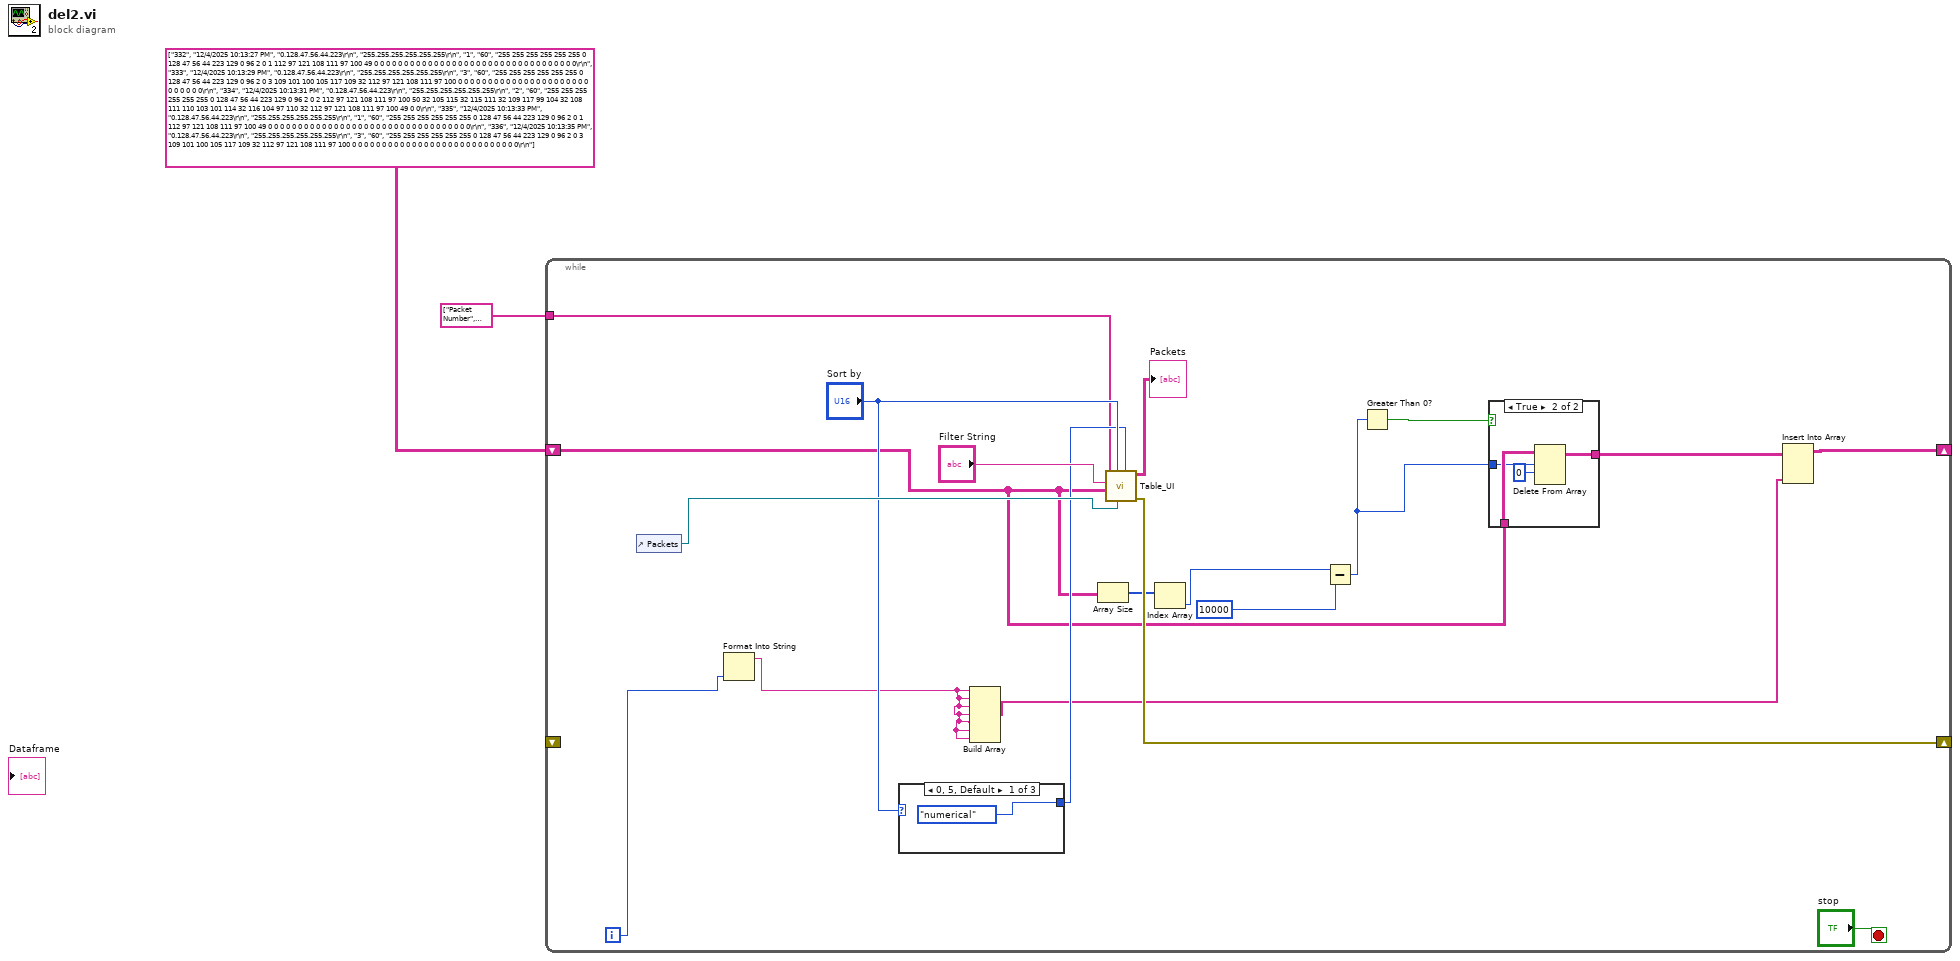
[diagram p0: block diagram]
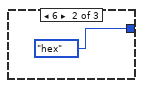
[diagram p2: hidden frame]
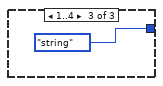
[diagram p3: hidden frame]
diagram:
  n1 = while {
    shift-right: [w21] -> _
    shift-left: _ -> [_]
    shift-right: [w20] -> _
    shift-left: string[][] [["332", "12/4/2025 10:13:27 PM", "0.128.47.56.44.223\r\n", "255.255.255.255.255.255\r\n", "1", "60", "255 255 255 255 255 255 0 128 47 56 44 223 129 0 96 2 0 1 112 97 121 108 111 97 100 49 0 0 0 0 0 0 0 0 0 0 0 0 0 0 0 0 0 0 0 0 0 0 0 0 0 0 0 0 0 0 0 0 0 0\r\n"], ["333", "12/4/2025 10:13:29 PM", "0.128.47.56.44.223\r\n", "255.255.255.255.255.255\r\n", "3", "60", "255 255 255 255 255 255 0 128 47 56 44 223 129 0 96 2 0 3 109 101 100 105 117 109 32 112 97 121 108 111 97 100 0 0 0 0 0 0 0 0 0 0 0 0 0 0 0 0 0 0 0 0 0 0 0 0 0 0 0 0\r\n"], ["334", "12/4/2025 10:13:31 PM", "0.128.47.56.44.223\r\n", "255.255.255.255.255.255\r\n", "2", "60", "255 255 255 255 255 255 0 128 47 56 44 223 129 0 96 2 0 2 112 97 121 108 111 97 100 50 32 105 115 32 115 111 32 109 117 99 104 32 108 111 110 103 101 114 32 116 104 97 110 32 112 97 121 108 111 97 100 49 0 0\r\n"], ["335", "12/4/2025 10:13:33 PM", "0.128.47.56.44.223\r\n", "255.255.255.255.255.255\r\n", "1", "60", "255 255 255 255 255 255 0 128 47 56 44 223 129 0 96 2 0 1 112 97 121 108 111 97 100 49 0 0 0 0 0 0 0 0 0 0 0 0 0 0 0 0 0 0 0 0 0 0 0 0 0 0 0 0 0 0 0 0 0 0\r\n"], ["336", "12/4/2025 10:13:35 PM", "0.128.47.56.44.223\r\n", "255.255.255.255.255.255\r\n", "3", "60", "255 255 255 255 255 255 0 128 47 56 44 223 129 0 96 2 0 3 109 101 100 105 117 109 32 112 97 121 108 111 97 100 0 0 0 0 0 0 0 0 0 0 0 0 0 0 0 0 0 0 0 0 0 0 0 0 0 0 0 0\r\n"]] -> [w7]
    tunnel: string[] ["Packet Number", "Timestamp", "Source", "Destination", "Protocol", "Length", "Data"] ("Headers") -> [w8]
    i -> [w4]
    stop <- "stop" stop-if-true
    n2 = control-ref of="Packets"() -> (w19:refnum<vi>)
    n3 = Format Into String(w4) -> (resulting string=w3:string)  [unwired: 3 in, 1 out]
    n4 = case shown="0, 5, Default" "Sort by" {
      tunnel: [enum16{"numerical", "hex", "string"}."numerical" ("Sort Type") enum16{"numerical", "hex", "string"}."hex" ("Sort Type") enum16{"numerical", "string", "hex"}."string" ("Sort Type")] -> w9
      frame 0, 5, Default {
      }
      frame 6 {
      }
      frame 1..4 {
      }
    }
    n5 = Build Array(w3, w3, w3, w3, w3, w3, w3) -> (w5:string[])
    n6 = Array Size(array=w7) -> (size(s)=w16:i32[])
    n7 = call "Table_UI.vi"("Sort Type"=w9, "Table Control Reference"=w19, "Sort by"="Sort by", "Prefiltered Data"=w7, "Filter String"="Filter String", "Headers"=w8) -> ("Error Out"=w21:errorcluster, "Table Control"=→"Packets":string[][])  [unwired: 4 in]
    n8 = Index Array(array=w16) -> (element=w14:i32)  [unwired: 1 in]
    n9 = Subtract(x=w14, y=10000) -> (x-y=w11:i32)
    n10 = Greater Than 0?(x=w11) -> (x > 0?=w12:bool)
    n11 = case shown="True" w12 {
      tunnel: w7 -> [w25 w29]
      tunnel: [w25 w28] -> w15
      tunnel: w11 -> [_ w27]
      frame False {
      }
      frame True {
        n12 = Delete From Array(array=w29, length=w27, index (row)=0) -> (array with subset deleted=w28:string[][])  [unwired: 1 in, 1 out]
      }
    }
    n13 = Insert Into Array(array=w15, new element=w5) -> (w20:string[][])  [unwired: 2 in]
  }
